vi "Create RIO Data Files.vi"(6 "Serial Numbers":string[](array[string]), 8 "Base Filename":string, 9 "Base Filepath":path, 10 "File Index In":i32, 11 "Anomaly Filepath In":path) -> (1 "Current Filepath":path, 2 "File Index Out":i32, 3 "Anomaly Filepath Out":path)   [LabVIEW 2013]
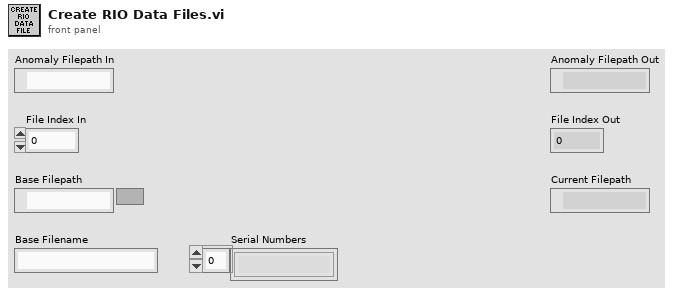
[diagram p1: front panel]
types:
  T1 = enum16{"open", "replace", "create", "open or create", "replace or create", "replace or create with confirmation"}
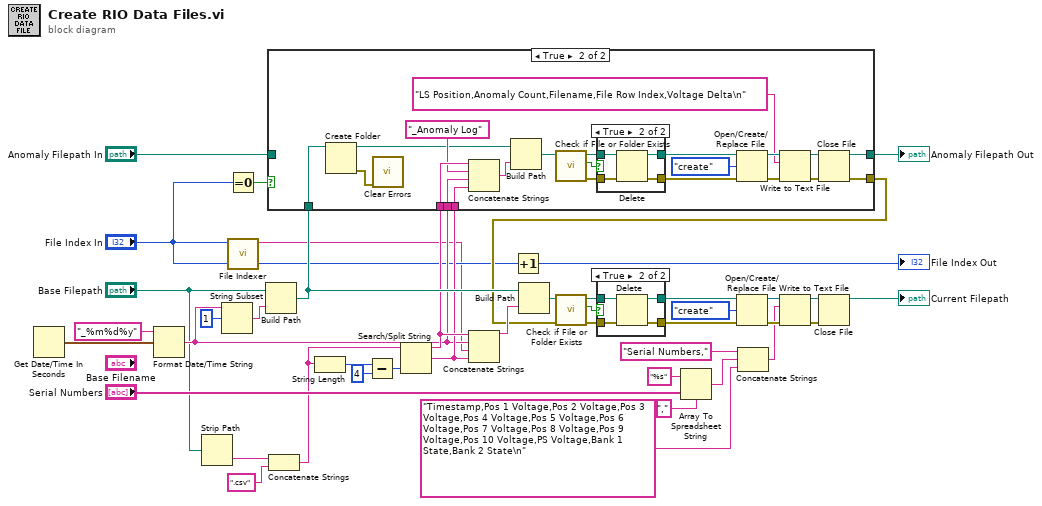
[diagram p0: block diagram]
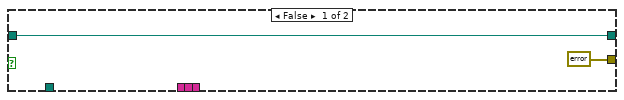
[diagram p2: hidden frame]
diagram:
  n1 = Get Date/Time In Seconds() -> (seconds since 1Jan1904=w19:timestamp)
  n2 = Format Date/Time String(time format string (%c)="_%m%d%y", seconds (now)=w19) -> (date/time string=w10:string)  [unwired: 1 in]
  n3 = Strip Path(path="Base Filepath") -> (name=w5:string)  [unwired: 1 out]
  n4 = String Subset(string=w10, offset (0)=1) -> (substring=w9:string)  [unwired: 1 in]
  n5 = Equal To 0?(x="File Index In") -> (x = 0?=w12:bool)
  n6 = call "File Indexer.vi"("File Index In"="File Index In") -> ("File Indicator Out"=w1:string)  [unwired: 10 in]
  n7 = Build Path(base path="Base Filepath", name or relative path=w9) -> (appended path=w16:path)
  n8 = Concatenate Strings(w5, ".csv" ("string")) -> (w3:string)
  n9 = String Length(string=w3) -> (length=w22:i32)
  n10 = Subtract(x=w22, y=4) -> (x-y=w20:i32)
  n11 = Search/Split String(string=w3, offset (0)=w20) -> (substring before match=w15:string, match + rest of string=w14:string)  [unwired: 1 in, 1 out]
  n12 = case shown="True" w12 {
    tunnel: w16 -> [_ w47]
    tunnel: w15 -> [_ w65]
    tunnel: w14 -> [_ w64]
    tunnel: w10 -> [_ w63]
    tunnel: [w44 w61] -> w13
    tunnel: "Anomaly Filepath In" -> [w44 _]
    tunnel: [errorcluster {"status"=FALSE, "code"=0, "source"=""} ("error out") w48] -> w7
    frame False {
    }
    frame True {
      n13 = Create Folder(path (use dialog)=w47) -> (created path=w46:path, error out=w45:errorcluster)  [unwired: 2 in, 1 out]
      n14 = call <vilib>:"Clear Errors.vi"("error in (no error)"=w45) -> ()  [unwired: 6 in, 1 out]
      n15 = Concatenate Strings(w65, "_Anomaly Log" ("string"), w63, w64) -> (w66:string)
      n16 = Build Path(base path=w46, name or relative path=w66) -> (appended path=w50:path)
      n17 = call <vilib>:"Check if File or Folder Exists.vi"("path"=w50) -> ("error out"=w52:errorcluster, "file or folder exists?"=w60:bool, "dup path"=w59:path)  [unwired: 8 in]
      n18 = case shown="True" w60 {
        tunnel: w59 -> [w68 w72]
        tunnel: [w68 w71] -> w53
        tunnel: w52 -> [w67 w70]
        tunnel: [w67 w69] -> w51
        frame False {
        }
        frame True {
          n19 = Delete(path (use dialog)=w72, error in=w70) -> (deleted path=w71:path, error out=w69:errorcluster)  [unwired: 3 in, 1 out]
        }
      }
      n20 = Open/Create/Replace File(file path (use dialog)=w53, error in=w51, operation (0:open)=T1."create") -> (refnum out=w57:refnum<file>, error out=w55:errorcluster)  [unwired: 3 in, 1 out]
      n21 = Write to Text File(file (use dialog)=w57, text="LS Position,Anomaly Count,Filename,File Row Index,Voltage Delta\n", error in=w55) -> (refnum out=w58:refnum<file>, error out=w56:errorcluster)  [unwired: 1 in, 1 out]
      n22 = Close File(refnum=w58, error in=w56) -> (path=w61:path, error out=w48:errorcluster)
    }
  }
  "Anomaly Filepath Out" <- w13
  n23 = Concatenate Strings(w15, w10, w1, w14) -> (w17:string)
  n24 = Increment(x="File Index In") -> (x+1=→"File Index Out":i32)
  n25 = Build Path(base path=w16, name or relative path=w17) -> (appended path=w26:path)
  n26 = call <vilib>:"Check if File or Folder Exists.vi"("error in (no error)"=w7, "path"=w26) -> ("error out"=w40:errorcluster, "file or folder exists?"=w27:bool, "dup path"=w28:path)  [unwired: 7 in]
  n27 = case shown="True" w27 {
    tunnel: w28 -> [w74 w78]
    tunnel: [w74 w77] -> w39
    tunnel: w40 -> [w73 w76]
    tunnel: [w73 w75] -> w41
    frame False {
    }
    frame True {
      n28 = Delete(path (use dialog)=w78, error in=w76) -> (deleted path=w77:path, error out=w75:errorcluster)  [unwired: 3 in, 1 out]
    }
  }
  n29 = Array To Spreadsheet String(delimiter (Tab)=",", array="Serial Numbers", 3:"%s" ("format string")) -> (spreadsheet string=w29:string)
  n30 = Open/Create/Replace File(file path (use dialog)=w39, error in=w41, operation (0:open)=T1."create") -> (refnum out=w35:refnum<file>, error out=w37:errorcluster)  [unwired: 3 in, 1 out]
  n31 = Concatenate Strings("Serial Numbers," ("string"), w29, "Timestamp,Pos 1 Voltage,Pos 2 Voltage,Pos 3 Voltage,Pos 4 Voltage,Pos 5 Voltage,Pos 6 Voltage,Pos 7 Voltage,Pos 8 Voltage,Pos 9 Voltage,Pos 10 Voltage,PS Voltage,Bank 1 State,Bank 2 State\n") -> (w32:string)
  n32 = Write to Text File(file (use dialog)=w35, text=w32, error in=w37) -> (refnum out=w34:refnum<file>, error out=w36:errorcluster)  [unwired: 1 in, 1 out]
  n33 = Close File(refnum=w34, error in=w36) -> (path=→"Current Filepath":path)  [unwired: 1 out]
